vi "ConfirmFile.vi"(4 "Error In":errorcluster, 5 "Filename IN":string, 6 "Run uninterrupted?":bool, 7 "Pathname IN":string) -> (0 "Error Out":errorcluster, 1 "Run Number":i32, 2 "comments OUT":string, 3 "Filename:":string)   [LabVIEW 2013]
uses:
  globals/QC_RunInformation.vi
panel:
  in  "enter comments:":string
  out "Pathname":string
  out "Folder already existed":bool
  in  "stop":bool
  # "Saving Data File"
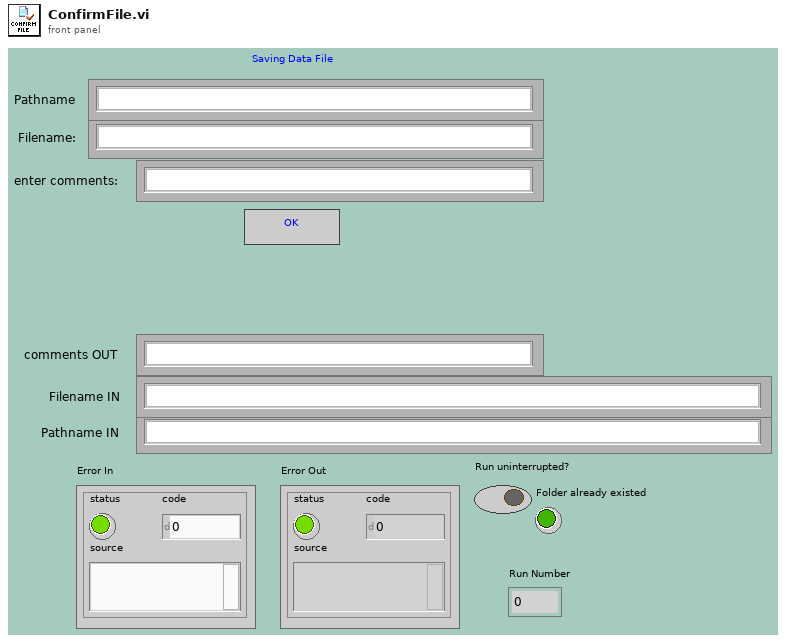
[diagram p1: front panel]
types:
  T1 = cluster{"Sensor Serial No.:":string, "Wafer:":string, "Batch:":string, "Manufacturer:":string, "Device Category:":string, "Database Serial No.:":string, "Date Initiated:":string, "Time Initiated:":string, "Test":string, "Probeplan used:":string, "End of Run comment:":string, "User:":string, "Vbias SMU":string, "LCR":string, "Test SMU":string, "Test DMM":string}
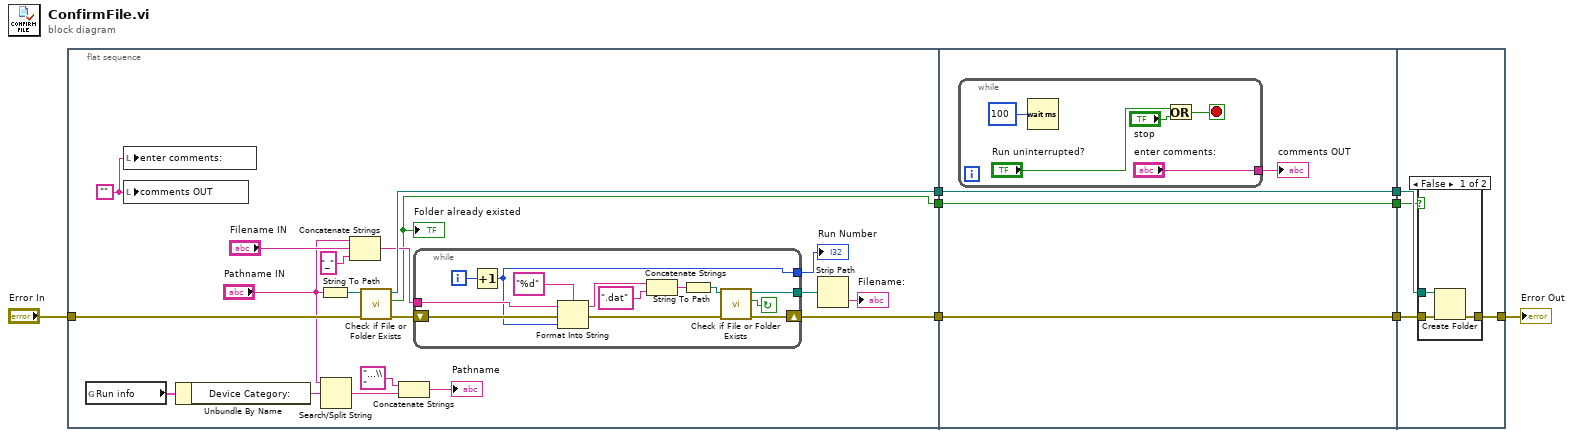
[diagram p0: block diagram]
diagram:
  n1 = flat-sequence {
    tunnel: "Error In" -> [w27]
    tunnel: [w22] -> w5
    tunnel: [w25] -> w4
    tunnel: [w20] -> w2
    tunnel: [w44] -> w6
    tunnel: w5 -> [w44]
    tunnel: w4 -> [w43]
    tunnel: [w43] -> w3
    tunnel: w2 -> [w42]
    tunnel: [w42] -> w1
    tunnel: [w53] -> w7
    tunnel: w6 -> [w52]
    tunnel: w3 -> [w51]
    tunnel: w1 -> [w50]
    frame #0 {
      w9 = ""
      n2 = global read "QC_RunInformation.vi" "Run info"() -> (w15:T1)
      n3 = local write "enter comments:"(w9) -> ()
      n4 = local write "comments OUT"(w9) -> ()
      n5 = Unbundle By Name(w15) -> ("Device Category:"=w14:string)
      n6 = String To Path(string="Pathname IN") -> (path=w26:path)
      n7 = Search/Split String(string="Pathname IN", search string/char (-)=w14) -> (match + rest of string=w12:string)  [unwired: 1 in, 2 out]
      n8 = Concatenate Strings("Pathname IN", "Filename IN", "_") -> (w21:string)
      n9 = call <vilib>:"Check if File or Folder Exists.vi"("error in (no error)"=w27, "path"=w26) -> ("error out"=w23:errorcluster, "file or folder exists?"=w20:bool, "dup path"=w25:path)  [unwired: 7 in]
      "Folder already existed" <- w20
      n10 = Concatenate Strings("...\\", w12) -> (→"Pathname":string)
      n11 = while {
        shift-right: [w39] -> w22
        shift-left: w23 -> [w34]
        tunnel: w21 -> [w37]
        tunnel: [w32] -> w18
        tunnel: [w28] -> w10
        i -> [w38]
        stop <- w40 continue-if-true
        n12 = Increment(x=w38) -> (x+1=w28:i32)
        n13 = Format Into String(format string="%d", initial string=w37, error in=w34, w28) -> (resulting string=w31:string, error out=w33:errorcluster)
        n14 = Concatenate Strings(w31, ".dat") -> (w29:string)
        n15 = String To Path(string=w29) -> (path=w35:path)
        n16 = call <vilib>:"Check if File or Folder Exists.vi"("error in (no error)"=w33, "path"=w35) -> ("error out"=w39:errorcluster, "file or folder exists?"=w40:bool, "dup path"=w32:path)  [unwired: 7 in]
      }
      "Run Number" <- w10
      n17 = Strip Path(path=w18) -> (name=→"Filename:":string)  [unwired: 1 out]
    }
    frame #1 {
      n18 = while {
        tunnel: ["enter comments:"] -> w41
        stop <- w46 stop-if-true
        n19 = Wait (ms)(milliseconds to wait=u32 100) -> ()  [unwired: 1 out]
        n20 = Or(x="Run uninterrupted?", y="stop") -> (x .or. y?=w46:bool)
      }
      "comments OUT" <- w41
    }
    frame #2 {
      n21 = case shown="False" w50 {
        tunnel: w52 -> [w56 w57]
        tunnel: w51 -> [w55 _]
        tunnel: [w54 w57] -> w53
        frame False {
          n22 = Create Folder(path (use dialog)=w55, error in=w56) -> (error out=w54:errorcluster)  [unwired: 1 in, 2 out]
        }
        frame True {
        }
      }
    }
  }
  "Error Out" <- w7
